vi "write_log_metadata.vi"(8 "error in (no error)":errorcluster, 10 "data":variant, 11 "scan_hdf5_log in":refnum<class "scan_2d_hdf5_log.lvclass">) -> (0 "error out":errorcluster, 3 "scan_hdf5_log out":refnum<class "scan_2d_hdf5_log.lvclass">)   [LabVIEW 2015, in "scan_2d_hdf5_log.lvclass"]
uses:
  scan_2d_hdf5_log.lvclass
  scan_2d_hdf5_log.lvclass/scan_2d_hdf5_log.ctl
  <vilib>/UPVI/lvhdf5/attribute.llb/Simple H5Awrite (Variant).vi
  <vilib>/UPVI/lvhdf5/attribute.llb/LVH5A Operation.ctl
  <vilib>/UPVI/lvhdf5/attribute.llb/Simple H5Awrite.xnode
  <vilib>/UPVI/lvhdf5/library.llb/HDF5 Ref.ctl
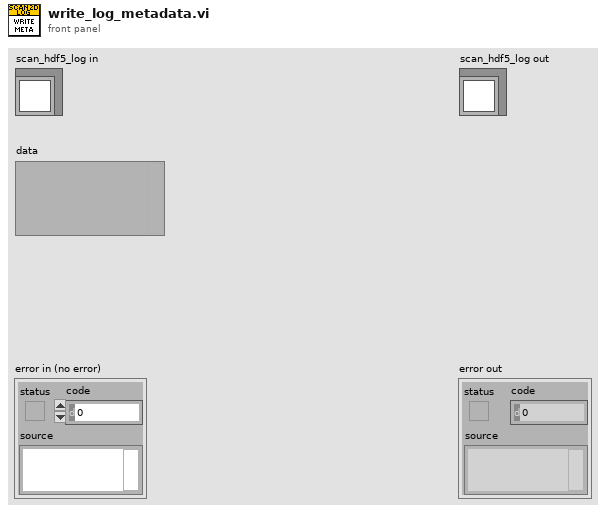
[diagram p1: front panel]
types:
  T1 = typedef "LVH5A Operation.ctl" = enum16{"open", "replace", "create", "open or create", "create or replace", "create or replace with confirmation"}
  T2 = typedef "data_types_tdef.ctl" = enum16{"0D", "1D", "2D"}
  T3 = typedef "HDF5 Ref.ctl" = refnum<k1>
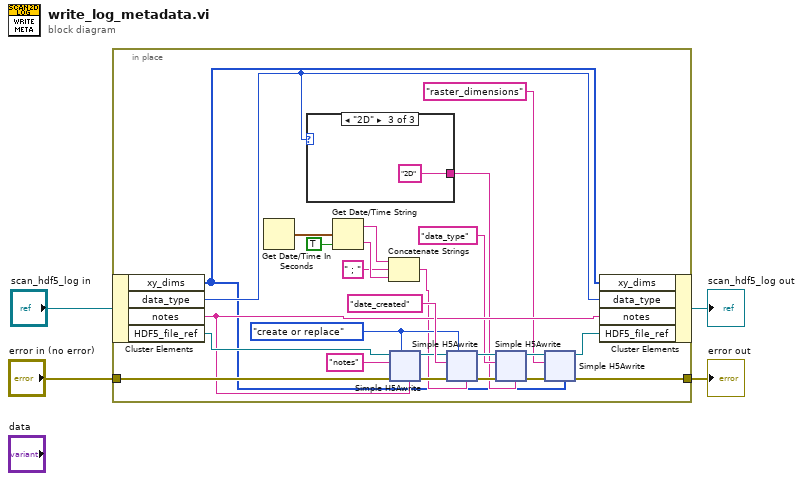
[diagram p0: block diagram]
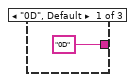
[diagram p2: hidden frame]
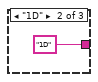
[diagram p3: hidden frame]
diagram:
  n1 = in-place {
    in-place-border: "error in (no error)" -> [w27]
    in-place-border: [w7] -> w1
    w22 = LVH5A_Operation."create or replace" ("operation (open or create)")
    n2 = in-place-cluster #1("scan_hdf5_log in") -> ("xy_dims"=w5:u32[], "data_type"=w11:T2, "notes"=w24:string, "HDF5_file_ref"=w29:T3)
    n3 = Get Date/Time In Seconds() -> (seconds since 1Jan1904=w21:timestamp)
    n4 = case shown="\"2D\"" w11 {
      tunnel: ["0D" "1D" "2D"] -> w12
      frame "0D", Default {
      }
      frame "1D" {
      }
      frame "2D" {
      }
    }
    n5 = Get Date/Time String(seconds (now)=w21, want seconds? (F)=TRUE) -> (date string=w19:string, time string=w18:string)  [unwired: 1 in]
    n6 = Concatenate Strings(w19, " ; " ("string"), w18) -> (w16:string)
    n7 = xnode "Simple H5Awrite"("HDF5 Ref"=w29, "Name"="notes", "error in (no error)"=w27, "operation (open or create)"=w22, "Value"=w24) -> ("HDF5 Ref out"=w23:T3, "error out"=w26:errorcluster)
    n8 = xnode "Simple H5Awrite"("HDF5 Ref"=w23, "Name"="date_created", "error in (no error)"=w26, "operation (open or create)"=w22, "Value"=w16) -> ("HDF5 Ref out"=w14:T3, "error out"=w15:errorcluster)
    n9 = xnode "Simple H5Awrite"("HDF5 Ref"=w14, "Name"="data_type", "error in (no error)"=w15, "Value"=w12) -> ("HDF5 Ref out"=w10:T3, "error out"=w9:errorcluster)  [unwired: 1 in]
    n10 = xnode "Simple H5Awrite"("HDF5 Ref"=w10, "Name"="raster_dimensions", "error in (no error)"=w9, "Value"=w5) -> ("HDF5 Ref out"=w8:T3, "error out"=w7:errorcluster)  [unwired: 1 in]
    n11 = in-place-cluster #1("xy_dims"=w5, "data_type"=w11, "notes"=w24, "HDF5_file_ref"=w8) -> (→"scan_hdf5_log out":refnum<class "scan_2d_hdf5_log.lvclass">)
  }
  "error out" <- w1
